vi "BL_LoadFirmware.vi"(0 "Potentiostat Galvanostat in":refnum<class "Potentiostat Galvanostat.lvclass">, 5 "Channels":u8[](array[numeric]), 7 "Bin File (.bin)":string, 9 "Xilinx File (.xlx)":string, 11 "error in (no error)":errorcluster) -> (4 "Potentiostat Galvanostat out":refnum<class "Potentiostat Galvanostat.lvclass">, 6 "Channels":u8[](array[numeric]), 8 "Channel Error Codes":i32[](array[numeric]), 15 "error out":errorcluster)   [LabVIEW 2018, in "Potentiostat Galvanostat.lvclass"]
doc: "This function tests the communication speed between the library and the selected channel. \nNOTE: This function is for advanced user only."
uses:
  Potentiostat Galvanostat.lvclass
  Potentiostat Galvanostat.lvclass/Potentiostat Galvanostat.ctl
  BL_GetErrorMsg.vi
  <vilib>/Utility/error.llb/Error Cluster From Error Code.vi
panel:
  in  "Force Reload?":bool
  in  "Show Gauge?":bool
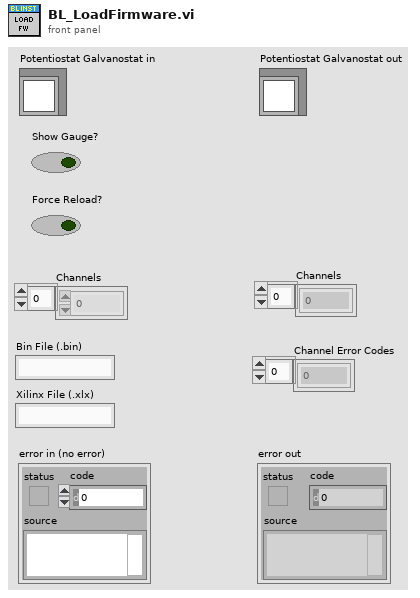
[diagram p1: front panel]
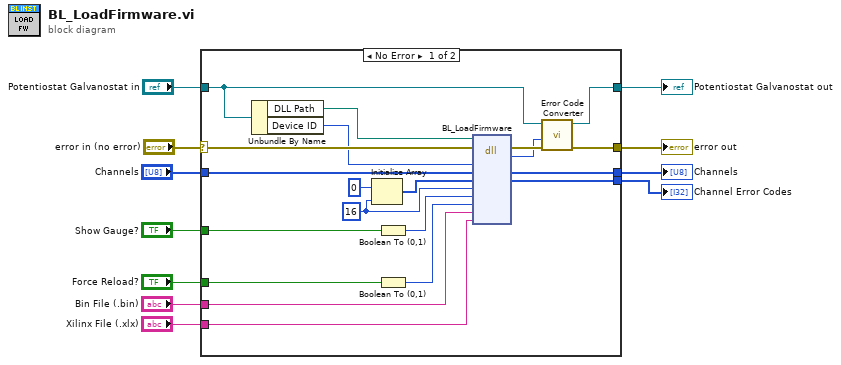
[diagram p0: block diagram]
diagram:
  n1 = case shown="No Error" "error in (no error)" {
    selector: "error in (no error)" -> [w19 w33]
    tunnel: [w15 w33] -> w10
    tunnel: [w13 w32] -> w8
    tunnel: "Potentiostat Galvanostat in" -> [w14 w32]
    tunnel: "Xilinx File (.xlx)" -> [w24 _]
    tunnel: "Bin File (.bin)" -> [w23 _]
    tunnel: "Force Reload?" -> [w22 _]
    tunnel: "Show Gauge?" -> [w21 _]
    tunnel: "Channels" -> [w20 _]
    tunnel: [w16 _] -> w2
    tunnel: [w12 _] -> w1
    frame No Error {
      w29 = 16 ("dimension size")
      n2 = Unbundle By Name(w14) -> ("DLL Path"=w18:path, "Device ID"=w17:i32)
      n3 = Initialize Array(0 ("element"), w29) -> (w30:i32[])
      n4 = Boolean To (0,1)(Boolean=w21) -> (0, 1=w28:i16)
      n5 = Boolean To (0,1)(Boolean=w22) -> (0, 1=w27:i16)
      n6 = dll-call lib="C:/Program Files (x86)/National Instruments/LabVIEW 2018/user.lib/EClib/EClib.*" fn="BL_LoadFirmware"(path in=w18, error in=w19, "Device ID"=w17, "Channels"=w20, "Channel Error Codes"=w30, "Channel Array Length"=w29, "Show Gauge?"=w28, "Force Reload?"=w27, "Bin File (.bin)"=w23, "Xilinx File (.xlx)"=w24) -> (error out=w26:errorcluster, "Error Code"=w25:i32, "Channels"=w12:u8[], "Channel Error Codes"=w16:i32[])  [unwired: 7 in, 1 out]
      n7 = call "Error Code Converter.vi"("error in (no error)"=w26, "Error Code"=w25, "Potentiostat Galvanostat in"=w14) -> ("error out"=w15:errorcluster, "Potentiostat Galvanostat out"=w13:refnum<class "Potentiostat Galvanostat.lvclass">)  [unwired: 7 in]
    }
    frame Error {
    }
  }
  "error out" <- w10
  "Potentiostat Galvanostat out" <- w8
  "Channel Error Codes" <- w2
  "Channels" <- w1
